vi "Set ICommunicate.vi"(8 "error in":errorcluster, 10 "ICommunicate":refnum<class "ICommunicate.lvclass">, 11 "Node Guard in":refnum<class "Node Guard.lvclass">) -> (0 "error out":errorcluster, 3 "Node Guard out":refnum<class "Node Guard.lvclass">)   [LabVIEW 2020, in "CANopen.lvlib" / "Network Management.lvlib" / "Node Guard.lvlib" / "Node Guard.lvclass"]
uses:
  Node Guard.lvclass
  Node Guard.lvclass/Node Guard.ctl
  HAL/Source/Interfaces/ICommunicate/ICommunicate.lvclass
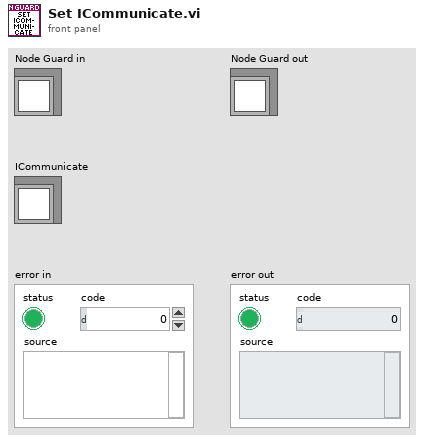
[diagram p1: front panel]
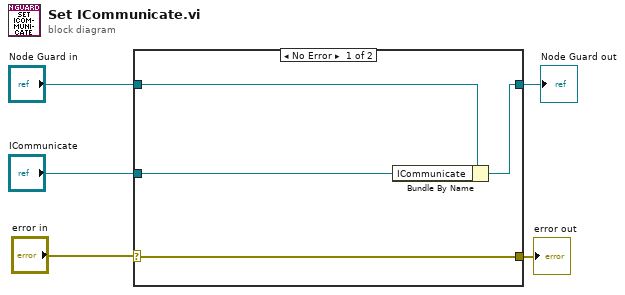
[diagram p0: block diagram]
diagram:
  n1 = case shown="No Error" "error in" {
    selector: "error in" -> [w9 w10]
    tunnel: [w9 w10] -> w2
    tunnel: [w7 w11] -> w4
    tunnel: "Node Guard in" -> [w8 w11]
    tunnel: "ICommunicate" -> [w6 _]
    frame No Error {
      n2 = Bundle By Name(cluster=w8, "ICommunicate"=w6) -> (w7:refnum<class "Node Guard.lvclass">)
    }
    frame Error {
    }
  }
  "error out" <- w2
  "Node Guard out" <- w4
